vi "sample for it.vi"(9 "Step 2":dbl=2.0, 10 "Stop 2":dbl=2.0, 11 "Start  2":dbl=1.0) -> (2 "Array 2":dbl[](array[numeric]) format="%#.1f", 3 "pointnumber 2":dbl)   [LabVIEW 2017]
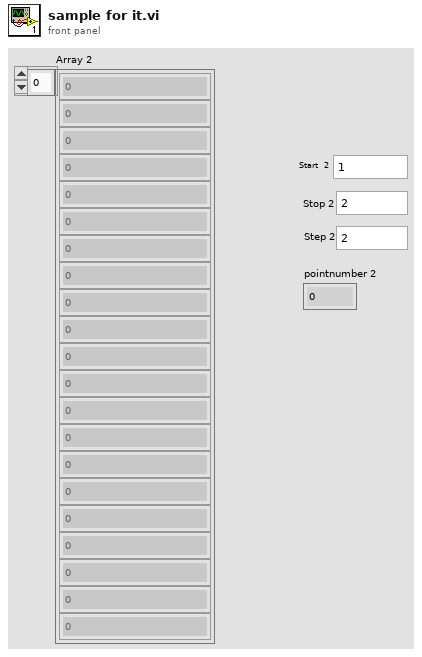
[diagram p1: front panel]
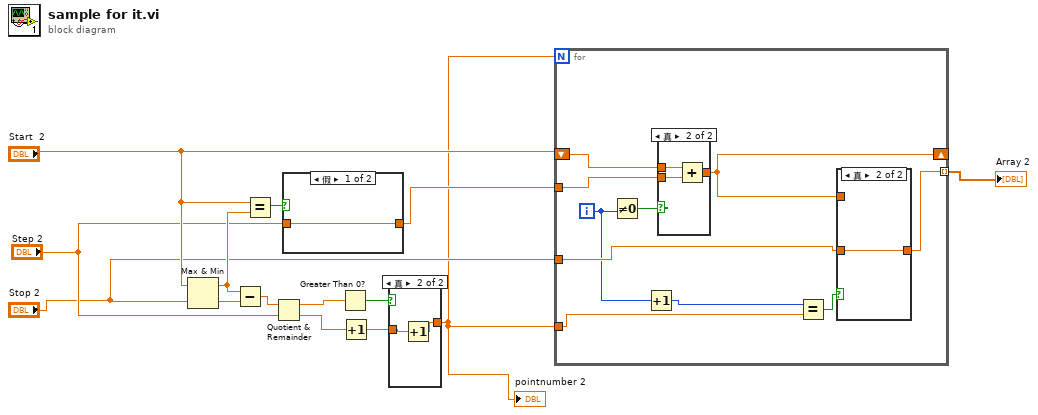
[diagram p0: block diagram]
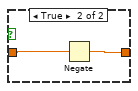
[diagram p3: hidden frame]
diagram:
  n1 = Max & Min(x="Start  2", y="Stop 2") -> (max(x,y)=w6:dbl, min(x,y)=w13:dbl)
  n2 = Subtract(x=w6, y=w13) -> (x-y=w14:dbl)
  n3 = Equal?(x="Start  2", y=w6) -> (x = y?=w12:bool)
  n4 = Quotient & Remainder(x=w14, y="Step 2") -> (x-y*floor(x/y)=w10:dbl, floor(x/y)=w8:dbl)
  n5 = case shown="假" w12 {
    tunnel: "Step 2" -> [w15 w17]
    tunnel: [w15 w16] -> w11
    frame False {
    }
    frame True {
      n6 = Negate(x=w17) -> (-x=w16:dbl)
    }
  }
  n7 = Greater Than 0?(x=w10) -> (x > 0?=w9:bool)
  n8 = Increment(x=w8) -> (x+1=w7:dbl)
  n9 = case shown="真" w9 {
    tunnel: [w18 w19] -> w1
    tunnel: w7 -> [w18 w20]
    frame False {
    }
    frame True {
      n10 = Increment(x=w20) -> (x+1=w19:dbl)
    }
  }
  "pointnumber 2" <- w1
  n11 = for {
    N: w1 -> [_]
    tunnel: w11 -> [w29]
    shift-right: [w26] -> _
    shift-left: "Start  2" -> [w30]
    tunnel: "Stop 2" -> [w25]
    tunnel: [w27] -> w5 mode=indexing
    tunnel: w1 -> [w22]
    i -> [w24]
    n12 = Not Equal To 0?(x=w24) -> (x != 0?=w28:bool)
    n13 = Increment(x=w24) -> (x+1=w23:i32)
    n14 = case shown="真" w28 {
      tunnel: w30 -> [w33 w36]
      tunnel: w29 -> [_ w35]
      tunnel: [w33 w34] -> w26
      frame False {
      }
      frame True {
        n15 = Add(x=w36, y=w35) -> (x+y=w34:dbl)
      }
    }
    n16 = Equal?(x=w23, y=w22) -> (x = y?=w21:bool)
    n17 = case shown="真" w21 {
      tunnel: w25 -> [_ w32]
      tunnel: [w31 w32] -> w27
      tunnel: w26 -> [w31 _]
      frame False {
      }
      frame True {
      }
    }
  }
  "Array 2" <- w5
